vi "XMLtoMacro.vi"(1 "XML File Path":path=path "C:/CuspControl/Cusp/1_Macros/Electrons/Catch/Barndoor_v6.mac") -> (0 "MacroSaveCluster":T3={"Instructions"=[{"Duration"=0.01, "Comment"="Initial state", "Steps"=1, "Edit Potential"=FALSE, "Output Bits"=[FALSE, FALSE, FALSE, FALSE, FALSE, FALSE, FALSE, FALSE, FALSE, FALSE, FALSE, FALSE, FALSE, FALSE, FALSE, FALSE, FALSE, FALSE, FALSE, FALSE, FALSE, FALSE, FALSE, FALSE, FALSE, FALSE, FALSE, FALSE, FALSE, FALSE, FALSE, FALSE, FALSE, FALSE, FALSE, FALSE, FALSE, FALSE], "Macro Path"=path "", "Potentials"=[0.1, 0.0, 0.0, 0.0, 0.0, 0.0, 0.0, 0.0, 0.0, 0.0, 0.0, 0.0, 0.0, 0.0, 0.0, 0.0], "Inherit?"=FALSE}, {"Duration"=0.05, "Comment"="Blocking potentials", "Steps"=500, "Edit Potential"=FALSE, "Output Bits"=[FALSE, FALSE, FALSE, FALSE, FALSE, FALSE, FALSE, FALSE, FALSE, FALSE, FALSE, FALSE, FALSE, FALSE, FALSE, FALSE, FALSE, FALSE, FALSE, FALSE, FALSE, FALSE, FALSE, FALSE, FALSE, FALSE, FALSE, FALSE, FALSE, FALSE, FALSE, FALSE, FALSE, FALSE, FALSE, FALSE, FALSE, FALSE], "Macro Path"=path "", "Potentials"=[-100.0, -25.0, -25.0, 0.0, -25.0, -25.0, -25.0, -25.0, -100.0, -100.0, 0.0, 0.0, 0.0, 0.0, 0.0, 0.0], "Inherit?"=FALSE}, {"Duration"=1.0, "Comment"="Wait 1 s", "Steps"=1, "Edit Potential"=FALSE, "Output Bits"=[FALSE, FALSE, FALSE, FALSE, FALSE, FALSE, FALSE, FALSE, FALSE, FALSE, FALSE, FALSE, FALSE, FALSE, FALSE, FALSE, FALSE, FALSE, FALSE, FALSE, FALSE, FALSE, FALSE, FALSE, FALSE, FALSE, FALSE, FALSE, FALSE, FALSE, FALSE, FALSE, FALSE, FALSE, FALSE, FALSE, FALSE, FALSE], "Macro Path"=path "", "Potentials"=[-100.0, -25.0, -25.0, 0.0, -25.0, -25.0, -25.0, -25.0, -100.0, -100.0, 0.0, 0.0, 0.0, 0.0, 0.0, 0.0], "Inherit?"=FALSE}, {"Duration"=0.05, "Comment"="Open US side", "Steps"=500, "Edit Potential"=FALSE, "Output Bits"=[FALSE, FALSE, FALSE, FALSE, FALSE, FALSE, FALSE, FALSE, FALSE, FALSE, FALSE, FALSE, FALSE, FALSE, FALSE, FALSE, FALSE, FALSE, FALSE, FALSE, FALSE, FALSE, FALSE, FALSE, FALSE, FALSE, FALSE, FALSE, FALSE, FALSE, FALSE, FALSE, FALSE, FALSE, FALSE, FALSE, FALSE, FALSE], "Macro Path"=path "", "Potentials"=[-49.0, -25.0, -25.0, 0.0, -25.0, -25.0, -25.0, -25.0, -100.0, -100.0, 0.0, 0.0, 0.0, 0.0, 0.0, 0.0], "Inherit?"=FALSE}, {"Duration"=2.0, "Comment"="Wait 2 s", "Steps"=1, "Edit Potential"=FALSE, "Output Bits"=[FALSE, FALSE, FALSE, FALSE, FALSE, FALSE, FALSE, FALSE, FALSE, FALSE, FALSE, FALSE, FALSE, FALSE, FALSE, FALSE, FALSE, FALSE, FALSE, FALSE, FALSE, FALSE, FALSE, FALSE, FALSE, FALSE, FALSE, FALSE, FALSE, FALSE, FALSE, FALSE, FALSE, FALSE, FALSE, FALSE, FALSE, FALSE], "Macro Path"=path "", "Potentials"=[-49.0, -25.0, -25.0, 0.0, -25.0, -25.0, -25.0, -25.0, -100.0, -100.0, 0.0, 0.0, 0.0, 0.0, 0.0, 0.0], "Inherit?"=FALSE}, {"Duration"=0.01, "Comment"="Close US side", "Steps"=1, "Edit Potential"=FALSE, "Output Bits"=[FALSE, FALSE, FALSE, FALSE, FALSE, FALSE, FALSE, FALSE, FALSE, FALSE, FALSE, FALSE, FALSE, FALSE, FALSE, FALSE, FALSE, FALSE, FALSE, FALSE, FALSE, FALSE, FALSE, FALSE, FALSE, FALSE, FALSE, FALSE, FALSE, FALSE, FALSE, FALSE, FALSE, FALSE, FALSE, FALSE, FALSE, FALSE], "Macro Path"=path "", "Potentials"=[-100.0, -25.0, -25.0, 0.0, -25.0, -25.0, -25.0, -25.0, -100.0, -100.0, 0.0, 0.0, 0.0, 0.0, 0.0, 0.0], "Inherit?"=FALSE}, {"Duration"=0.01, "Comment"="To u7", "Steps"=100, "Edit Potential"=FALSE, "Output Bits"=[FALSE, FALSE, FALSE, FALSE, FALSE, FALSE, FALSE, FALSE, FALSE, FALSE, FALSE, FALSE, FALSE, FALSE, FALSE, FALSE, FALSE, FALSE, FALSE, FALSE, FALSE, FALSE, FALSE, FALSE, FALSE, FALSE, FALSE, FALSE, FALSE, FALSE, FALSE, FALSE, FALSE, FALSE, FALSE, FALSE, FALSE, FALSE], "Macro Path"=path "", "Potentials"=[-100.0, -20.0, -20.0, 0.0, 0.0, 0.0, 0.0, -100.0, -100.0, -100.0, 0.0, 0.0, 0.0, 0.0, 0.0, 0.0], "Inherit?"=FALSE}, {"Duration"=0.01, "Comment"="To u7", "Steps"=100, "Edit Potential"=FALSE, "Output Bits"=[FALSE, FALSE, FALSE, FALSE, FALSE, FALSE, FALSE, FALSE, FALSE, FALSE, FALSE, FALSE, FALSE, FALSE, FALSE, FALSE, FALSE, FALSE, FALSE, FALSE, FALSE, FALSE, FALSE, FALSE, FALSE, FALSE, FALSE, FALSE, FALSE, FALSE, FALSE, FALSE, FALSE, FALSE, FALSE, FALSE, FALSE, FALSE], "Macro Path"=path "", "Potentials"=[-100.0, -100.0, -100.0, 0.0, 0.0, 0.0, 0.0, -100.0, -100.0, -100.0, 0.0, 0.0, 0.0, 0.0, 0.0, 0.0], "Inherit?"=FALSE}, {"Duration"=0.01, "Comment"="To u7", "Steps"=100, "Edit Potential"=FALSE, "Output Bits"=[FALSE, FALSE, FALSE, FALSE, FALSE, FALSE, FALSE, FALSE, FALSE, FALSE, FALSE, FALSE, FALSE, FALSE, FALSE, FALSE, FALSE, FALSE, FALSE, FALSE, FALSE, FALSE, FALSE, FALSE, FALSE, FALSE, FALSE, FALSE, FALSE, FALSE, FALSE, FALSE, FALSE, FALSE, FALSE, FALSE, FALSE, FALSE], "Macro Path"=path "", "Potentials"=[-100.0, -100.0, -100.0, 0.0, 100.0, 100.0, 100.0, -100.0, -100.0, -100.0, 0.0, 0.0, 0.0, 0.0, 0.0, 0.0], "Inherit?"=FALSE}, {"Duration"=0.01, "Comment"="To u7", "Steps"=100, "Edit Potential"=FALSE, "Output Bits"=[FALSE, FALSE, FALSE, FALSE, FALSE, FALSE, FALSE, FALSE, FALSE, FALSE, FALSE, FALSE, FALSE, FALSE, FALSE, FALSE, FALSE, FALSE, FALSE, FALSE, FALSE, FALSE, FALSE, FALSE, FALSE, FALSE, FALSE, FALSE, FALSE, FALSE, FALSE, FALSE, FALSE, FALSE, FALSE, FALSE, FALSE, FALSE], "Macro Path"=path "", "Potentials"=[-100.0, 0.0, 0.0, 0.0, 0.0, 100.0, 100.0, 0.0, 0.0, 0.0, 0.0, 0.0, 0.0, 0.0, 0.0, 0.0], "Inherit?"=FALSE}, {"Duration"=0.01, "Comment"="To u7", "Steps"=100, "Edit Potential"=FALSE, "Output Bits"=[FALSE, FALSE, FALSE, FALSE, FALSE, FALSE, FALSE, FALSE, FALSE, FALSE, FALSE, FALSE, FALSE, FALSE, FALSE, FALSE, FALSE, FALSE, FALSE, FALSE, FALSE, FALSE, FALSE, FALSE, FALSE, FALSE, FALSE, FALSE, FALSE, FALSE, FALSE, FALSE, FALSE, FALSE, FALSE, FALSE, FALSE, FALSE], "Macro Path"=path "", "Potentials"=[-100.0, 0.0, 0.0, 0.0, 0.0, 0.0, 100.0, 0.0, 0.0, 0.0, 0.0, 0.0, 0.0, 0.0, 0.0, 0.0], "Inherit?"=FALSE}], "Changes"=[[TRUE, TRUE], [FALSE, TRUE], [FALSE, FALSE], [FALSE, TRUE], [FALSE, FALSE], [FALSE, TRUE], [FALSE, TRUE], [FALSE, TRUE], [FALSE, TRUE], [FALSE, TRUE], [FALSE, TRUE]], "Macro Description"="Catch, including u10", "Total Time (s)"=3.17, "Samples per sec"=10000.0} {"Instructions"."Steps" min=1 max=100000 step=1; "Instructions"."Duration" min=0.001 step=0.001 format="%_6p"})   [LabVIEW 2018]
uses:
  MacroSaveCluster.ctl
  Instructions.ctl
  Executor Files/RT/Instruction.ctl
  MacroSaveCluster_legacy.ctl
  Instructions_legacy.ctl
  <vilib>/Utility/xml.llb/Read From XML File(string).vi
panel:
  in  "legacy prototype cluster":T1 {"Instructions"."Steps" min=1 max=100000 step=1; "Instructions"."Duration" min=0.001 step=0.001 format="%_6p"}
  in  "Reformat":bool=TRUE
  in  "prototype cluster":T3={"Instructions"=[], "Changes"=[], "Macro Description"="ERROR: Macro does not exist!", "Total Time (s)"=0.0, "Samples per sec"=0.0} {"Instructions"."Steps" min=1 max=100000 step=1; "Instructions"."Duration" min=0.001 step=0.001 format="%_6p"}
  # "0        2       4       6        8      10     12     14     16     18      20    22     24     26     28     30     32     34     36"
  # "0        2       4       6        8      10     12     14"
  # "0        2       4       6        8      10     12     14     16     18      20    22     24     26     28     30     32     34     36"
  # "0        2       4       6        8      10     12     14     16     18      20    22     24     26     28     30     32     34     36"
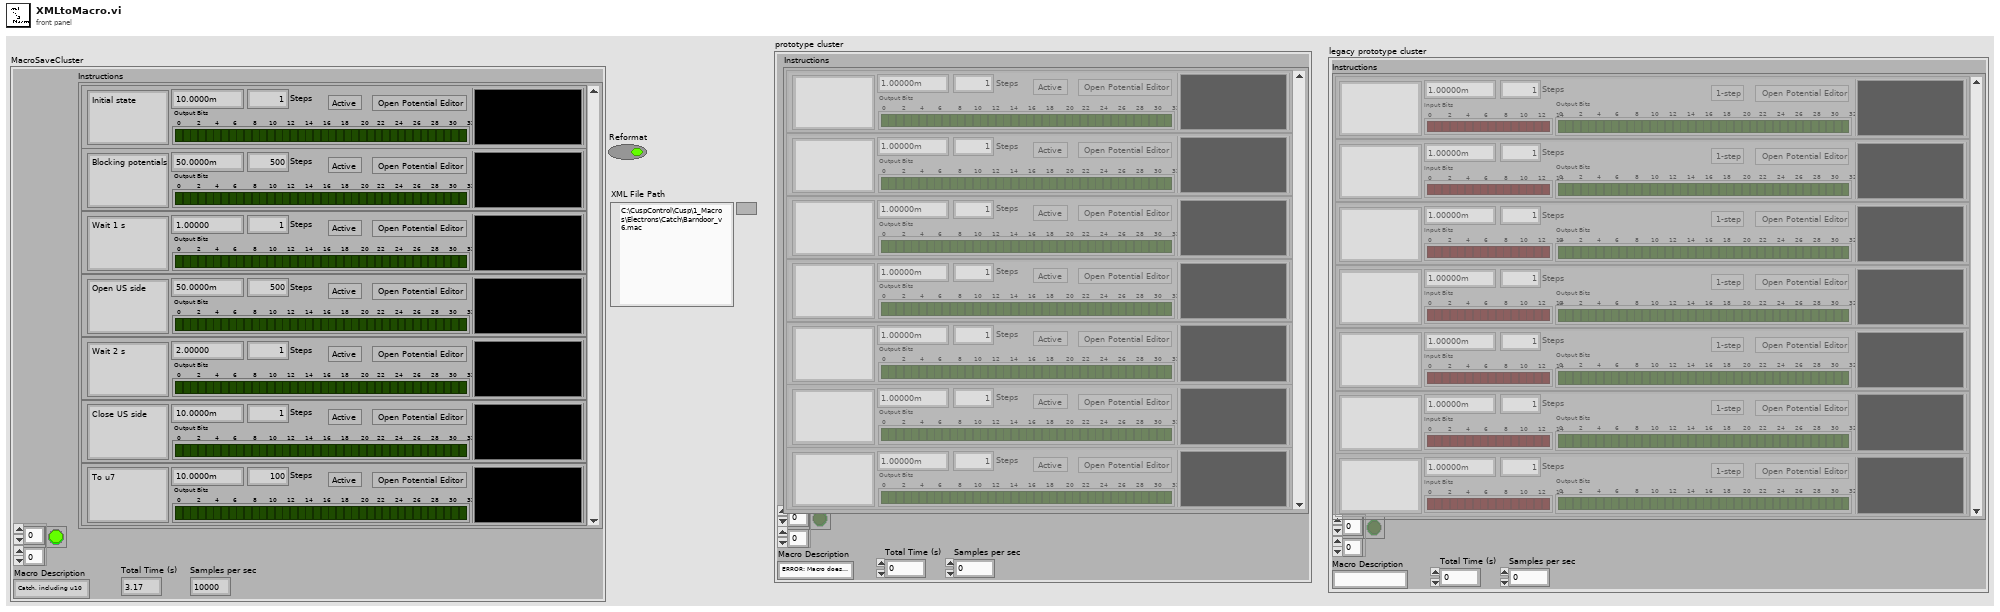
[diagram p1: front panel]
types:
  T1 = typedef "MacroSaveCluster_legacy.ctl" = cluster{"Instructions":T2, "Changes":bool[][], "Macro Description":string, "Total Time (s)":dbl, "Samples per sec":dbl}
  T2 = typedef "Instructions_legacy.ctl" = cluster{"Duration":dbl, "Comment":string, "Input Bits":bool[], "Steps":i32, "Edit Potential":bool, "Output Bits":bool[], "Macro Path":path, "Potentials":dbl[], "Ramp/Point":bool}[]
  T3 = typedef "MacroSaveCluster.ctl" = cluster{"Instructions":T4, "Changes":bool[][], "Macro Description":string, "Total Time (s)":dbl, "Samples per sec":dbl}
  T4 = typedef "Instructions.ctl" = T5[]
  T5 = typedef "Instruction.ctl" = cluster{"Duration":dbl, "Comment":string, "Steps":i32, "Edit Potential":bool, "Output Bits":bool[], "Macro Path":path, "Potentials":dbl[], "Inherit?":bool}
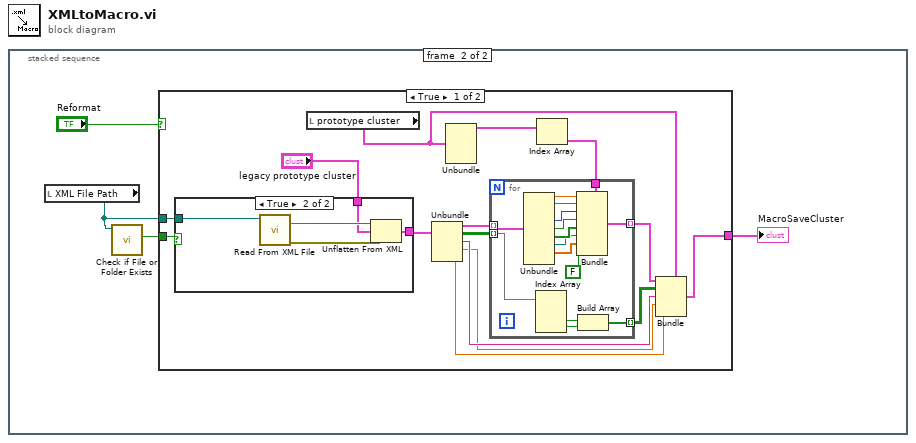
[diagram p0: block diagram]
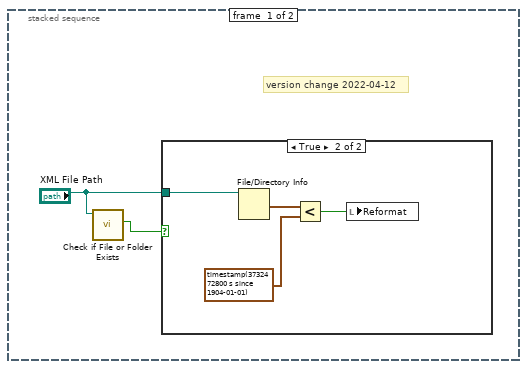
[diagram p2: hidden frame]
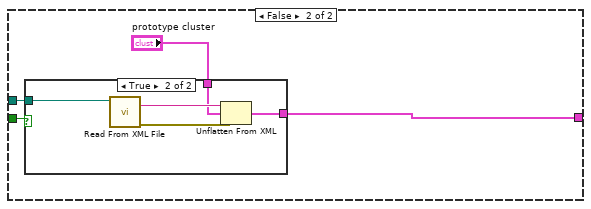
[diagram p5: hidden frame]
diagram:
  n1 = stacked-sequence {
    frame #0 {
      # "version change 2022-04-12"
      n2 = call <vilib>:"Check if File or Folder Exists.vi"("path"="XML File Path") -> ("file or folder exists?"=w1:bool)  [unwired: 8 in, 2 out]
      n3 = case shown="True" w1 {
        tunnel: "XML File Path" -> [_ w3]
        frame False {
        }
        frame True {
          n4 = File/Directory Info(path=w3) -> (last mod=w6:timestamp)  [unwired: 1 in, 6 out]
          n5 = Less?(x=w6, y=timestamp(3732472800 s since 1904-01-01) ("last mod")) -> (x < y?=w4:bool)
          n6 = local write "Reformat"(w4) -> ()
        }
      }
    }
    frame #1 {
      n7 = local read "XML File Path"() -> (w7:path)
      n8 = call <vilib>:"Check if File or Folder Exists.vi"("path"=w7) -> ("file or folder exists?"=w10:bool)  [unwired: 8 in, 2 out]
      n9 = case shown="True" "Reformat" {
        tunnel: w7 -> [w24 w49]
        tunnel: w10 -> [w23 w48]
        tunnel: [w11 w47] -> w8
        frame True {
          n10 = case shown="True" w23 {
            tunnel: w24 -> [_ w46]
            tunnel: "legacy prototype cluster" -> [w41 w43]
            tunnel: [w41 w42] -> w22
            frame False {
            }
            frame True {
              n11 = call-poly <vilib>:"Read From XML File.vi"("XML File Path"=w46) -> ("error out"=w44:errorcluster, "XML Elements"=w45:string)  [unwired: 8 in, 1 out]
              n12 = Unflatten From XML(xml string=w45, type=w43, error in (no error)=w44) -> (value=w42:T1)  [unwired: 1 out]
            }
          }
          n13 = local read "prototype cluster"() -> (w17:T3)
          n14 = Unbundle(w22) -> ("Instructions"=w21:T2, "Changes"=w20:bool[][], "Macro Description"=w14:string, "Total Time (s)"=w13:dbl, "Samples per sec"=w12:dbl)
          n15 = Unbundle(w17) -> ("Instructions"=w18:T4)  [unwired: 4 out]
          n16 = Index Array(array=w18) -> (element=w19:T5)  [unwired: 1 in]
          n17 = for {
            tunnel: w21 -> [w40] mode=indexing
            tunnel: w20 -> [w30] mode=indexing
            tunnel: w19 -> [w39]
            tunnel: [w27] -> w16 mode=indexing
            tunnel: [w26] -> w15 mode=indexing
            n18 = Unbundle(w40) -> ("Duration"=w38:dbl, "Comment"=w37:string, "Steps"=w36:i32, "Edit Potential"=w35:bool, "Output Bits"=w34:bool[], "Macro Path"=w33:path, "Potentials"=w32:dbl[])  [unwired: 2 out]
            n19 = Index Array(array=w30) -> (element #2=w29:bool, element #3=w28:bool)  [unwired: 3 in, 1 out]
            n20 = Bundle(cluster=w39, "Duration"=w38, "Comment"=w37, "Steps"=w36, "Edit Potential"=w35, "Output Bits"=w34, "Macro Path"=w33, "Potentials"=w32, "Inherit?"=FALSE) -> (w27:T5)
            n21 = Build Array(w29, w28) -> (w26:bool[])
          }
          n22 = Bundle(cluster=w17, "Instructions"=w16, "Changes"=w15, "Macro Description"=w14, "Total Time (s)"=w13, "Samples per sec"=w12) -> (w11:T3)
        }
        frame False {
          n23 = case shown="True" w48 {
            tunnel: w49 -> [_ w56]
            tunnel: "prototype cluster" -> [w51 w53]
            tunnel: [w51 w52] -> w47
            frame False {
            }
            frame True {
              n24 = call-poly <vilib>:"Read From XML File.vi"("XML File Path"=w56) -> ("error out"=w54:errorcluster, "XML Elements"=w55:string)  [unwired: 8 in, 1 out]
              n25 = Unflatten From XML(xml string=w55, type=w53, error in (no error)=w54) -> (value=w52:T3)  [unwired: 1 out]
            }
          }
        }
      }
      "MacroSaveCluster" <- w8
    }
  }
